vi "test1.vi"() -> ()   [LabVIEW 2020]
uses:
  <vilib>/Analysis/NI_AALBase.lvlib
  <vilib>/numeric/Random Number (Range) I64.vi
  <vilib>/DAQmx/create/channels.llb/DAQmx Create Channel (AI-Voltage-Basic).vi
  <vilib>/DAQmx/configure/timing.llb/DAQmx Timing (Implicit).vi
panel:
  in  "Terminate":bool
  in  "Choose image":bool
  out "XY Graph 3":cluster{"X":dbl[], "Y":dbl[]}[](graph)
  out "fit radius 3":dbl=0.3
  out "fit x-offset 3":dbl=0.1
  out "fit y-offset 3":dbl=0.2
  out "fit x-offset 2":dbl=0.1
  out "fit y-offset 2":dbl=0.2
  out "fit radius 2":dbl=0.3
  out "XY Graph 2":cluster{"X":dbl[], "Y":dbl[]}[](graph)
  out "Array 2":dbl[][](array[numeric])
  out "Time Stamp 2":timestamp format="%<%.6X\n%x>T"
  out "Time Stamp":timestamp format="%<%.6X\n%x>T"
  in  "x-offset":dbl=0.1
  in  "y-offset":dbl=0.2
  in  "radius":dbl=0.3
  in  "noise sigma":dbl=0.021 format="%.4f"
  out "XY Graph":cluster{"X":dbl[], "Y":dbl[]}[](graph)
  out "fit radius":dbl=0.3
  out "fit x-offset":dbl=0.1
  out "fit y-offset":dbl=0.2
  in  "loop terminate 2":bool
  out "led 2":bool
  in  "semaphore button":bool
  in  "semaphore terminate":bool
  out "led 1":bool
  out "Numeric 4":i32
  out "Cluster 3":cluster{"Numeric":dbl, "Numeric 2":dbl}
  out "Numeric 3":i32
  out "Numeric 2":i32
  out "Array":dbl[](array[numeric])
  out "Cluster 2":cluster{"Numeric 2":dbl, "Numeric 3":dbl}
  out "Cluster":cluster{"Numeric 2":dbl, "Numeric 3":dbl}
  in  "while terminate":bool
  out "cursor busy":bool
  in  "Ring":u16(ring) items=["12321"=0, "234"=1232, "343"=34343]
  out "Numeric":dbl
  in  "Cancel Button":bool
  in  "sw 3":bool
  in  "sw 2":bool
  out "Boolean 2":bool
  in  "sw":bool
  out "Boolean":bool
  out "num3":i32
  out "res":i32
  out "num2":i32
  out "num1":i32
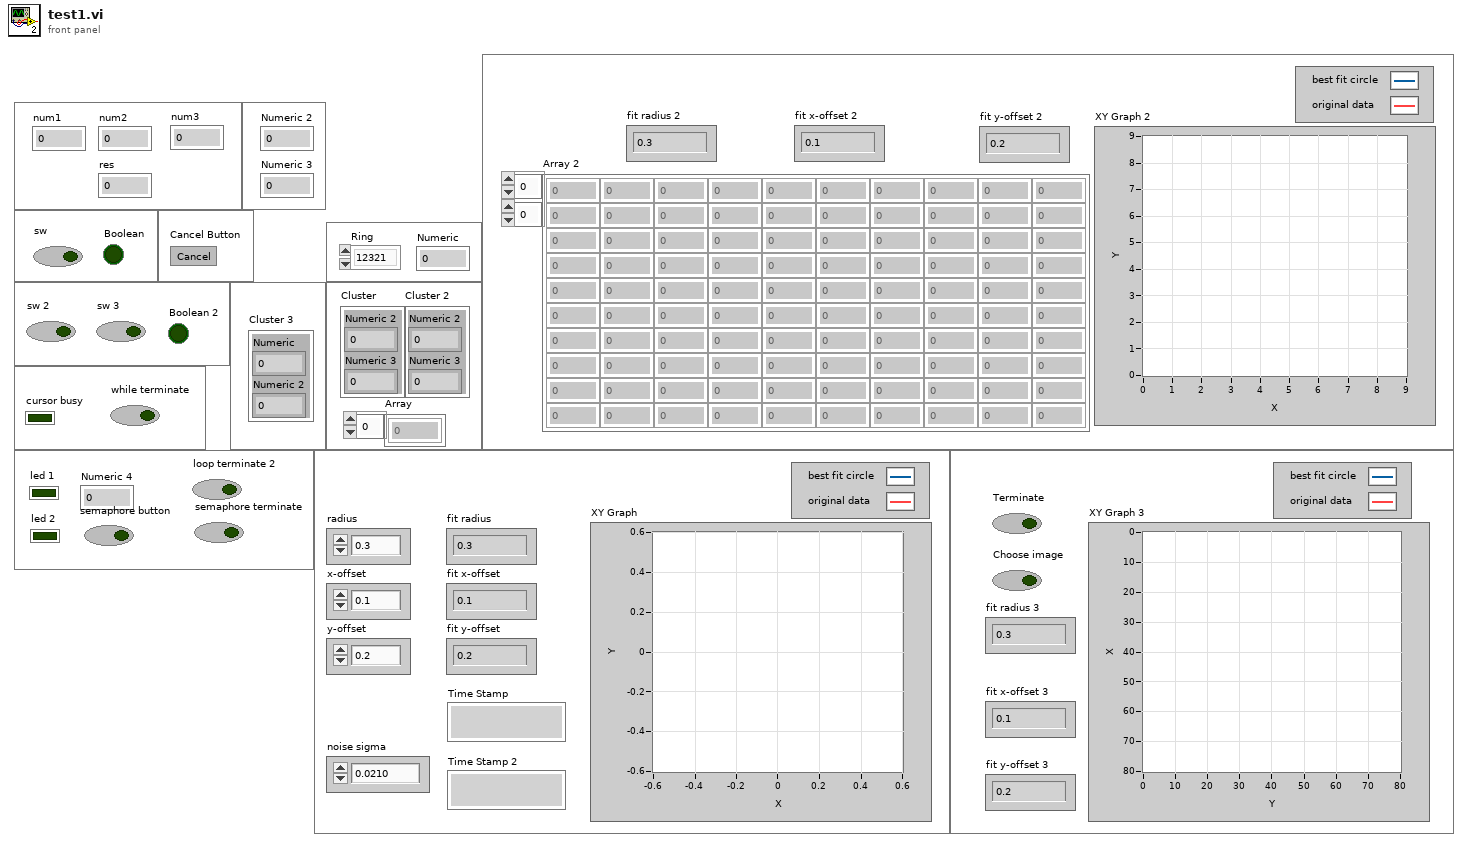
[diagram p1: front panel]
types:
  T1 = typedef "imagedata.ctl" = cluster{"image type":i32, "image depth":i32, "image":u8[], "mask":u8[], "colors":u32[], "Rectangle":cluster{"left":i16, "top":i16, "right":i16, "bottom":i16}}
  T2 = typedef "Semaphore RefNum" = refnum<k1>
  T3 = cluster{"[0]":i32, "[1]":i32, "[2]":i32, "[3]":i32, "[4]":i32, "[5]":i32, "[6]":i32, "[7]":i32, "[8]":i32}
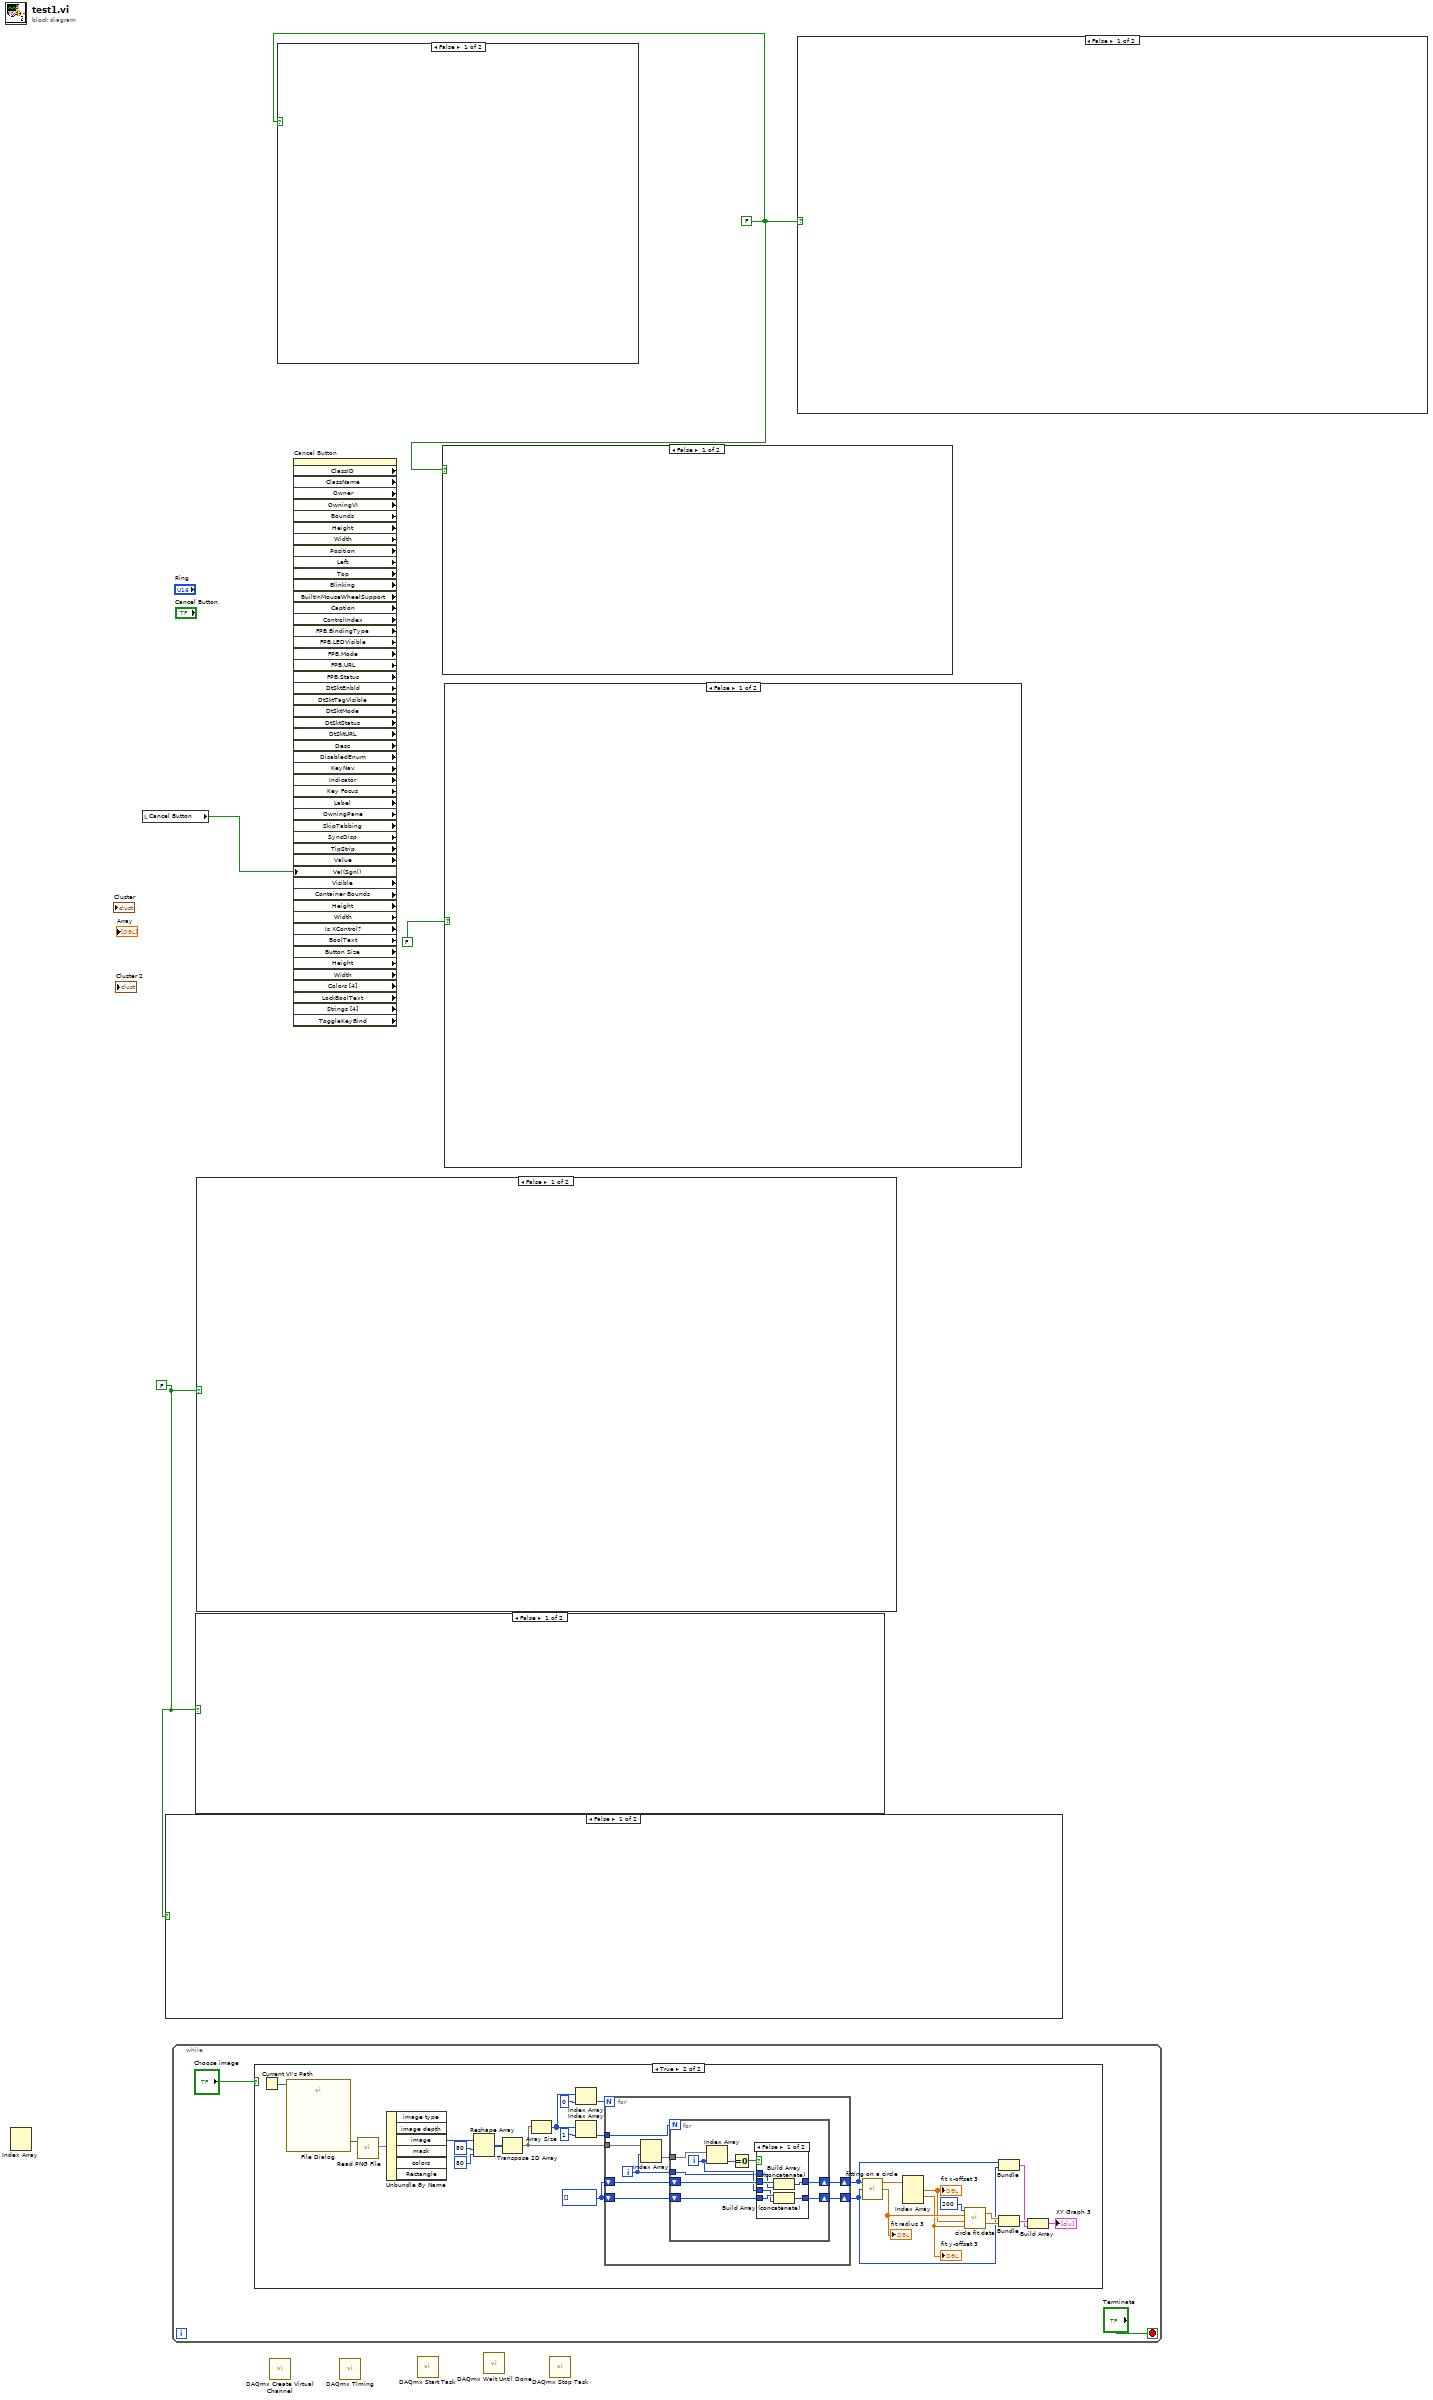
[diagram p0: block diagram]
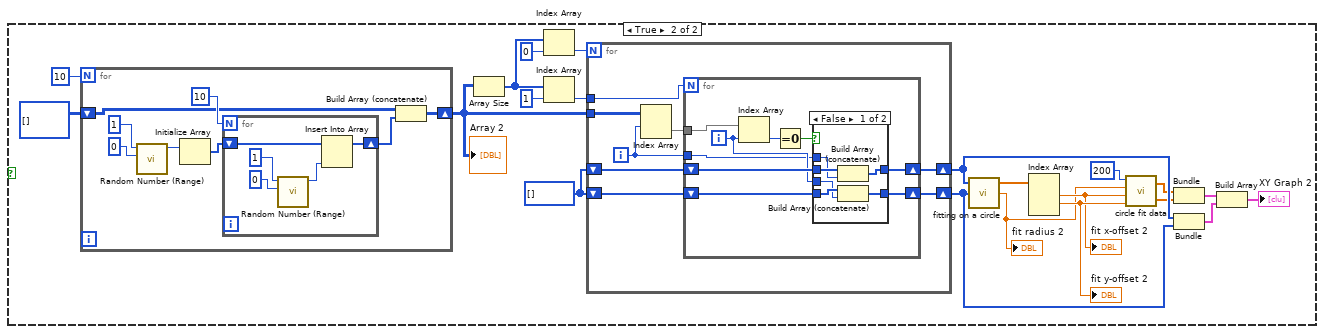
[diagram p4: hidden frame]
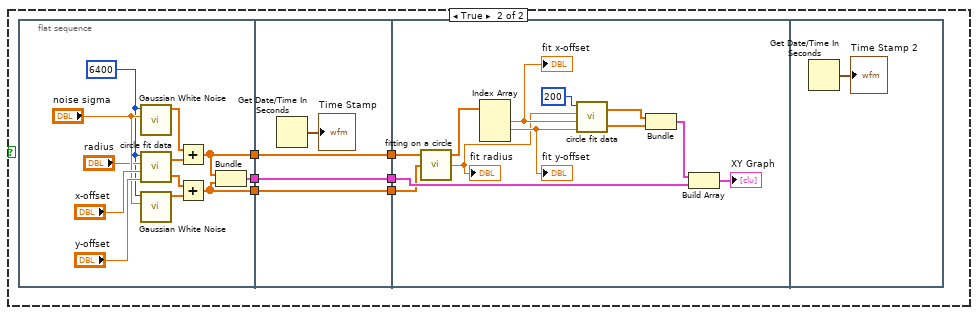
[diagram p6: hidden frame]
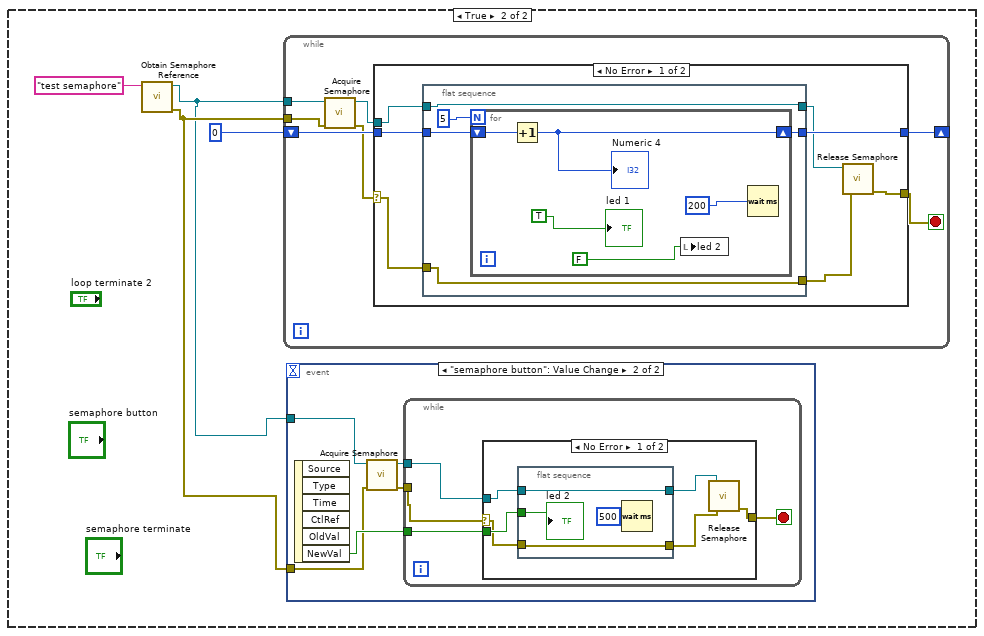
[diagram p7: hidden frame]
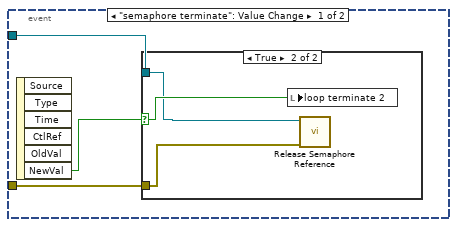
[diagram p8: hidden frame]
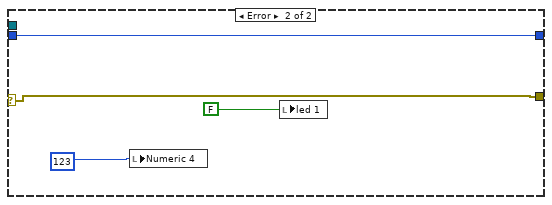
[diagram p11: hidden frame]
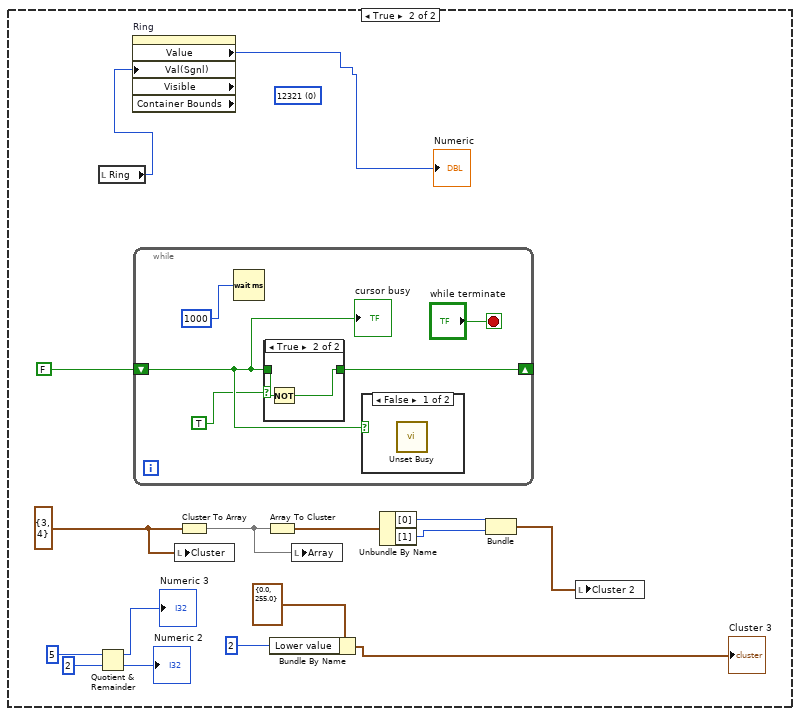
[diagram p12: hidden frame]
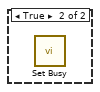
[diagram p14: hidden frame]
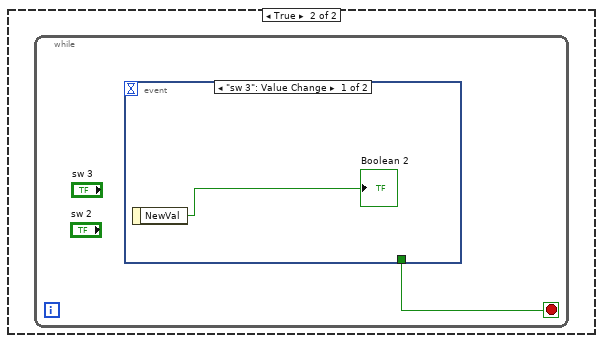
[diagram p15: hidden frame]
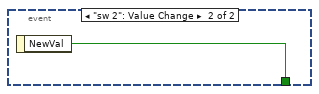
[diagram p16: hidden frame]
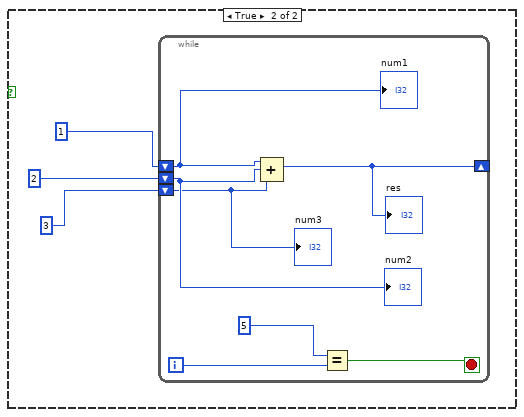
[diagram p17: hidden frame]
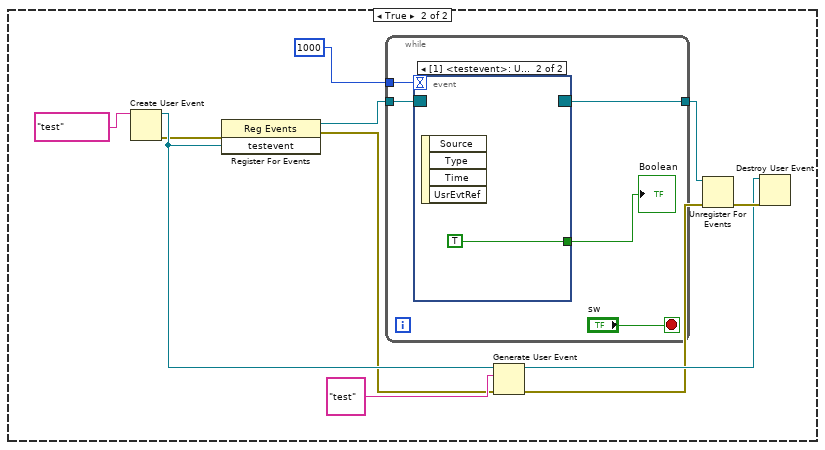
[diagram p18: hidden frame]
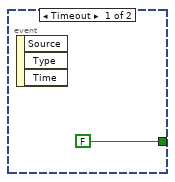
[diagram p19: hidden frame]
diagram:
  w1 = FALSE
  w4 = FALSE
  n1 = Index Array() -> ()  [unwired: 3 in, 2 out]
  n2 = local read "Cancel Button"() -> (w3:bool)
  n3 = case shown="False" w1 {
    frame False {
    }
    frame True {
      w7 = i32[] []
      n4 = for {
        N: 10 -> [_]
        shift-right: [w57] -> w21
        shift-left: i32[][] [] -> [w56]
        n5 = call-poly <vilib>:"Random Number (Range).vi"("lower bound (-100)"=0, "upper bound (100)"=1) -> ("number"=w53:i64)  [unwired: 9 in]
        n6 = Initialize Array(w53) -> (w52:i64[])  [unwired: 1 in]
        n7 = for {
          N: 10 -> [_]
          shift-right: [w59] -> w51
          shift-left: w52 -> [w60]
          n8 = call-poly <vilib>:"Random Number (Range).vi"("lower bound (-100)"=0, "upper bound (100)"=1) -> ("number"=w61:i64)  [unwired: 9 in]
          n9 = Insert Into Array(array=w60, new element=w61) -> (w59:i64[])  [unwired: 1 in]
        }
        n10 = Build Array (concatenate)(w56, w51) -> (w57:i64[][])
      }
      "Array 2" <- w21
      n11 = Array Size(array=w21) -> (size(s)=w25:i32[])
      n12 = Index Array(array=w25, index=0) -> (element=w23:i32)
      n13 = Index Array(array=w25, index=1) -> (element=w24:i32)
      n14 = for {
        N: w23 -> [_]
        tunnel: w24 -> [w33]
        shift-right: [w27] -> w15
        shift-left: w7 -> [w32]
        shift-right: [w26] -> w22
        shift-left: w7 -> [w31]
        tunnel: w21 -> [w30]
        i -> [w28]
        n15 = Index Array(array=w30, index (row)=w28) -> (element=w29:i64[])  [unwired: 1 in]
        n16 = for {
          N: w33 -> [_]
          shift-right: [w34] -> w27
          shift-left: w32 -> [w39]
          shift-right: [w38] -> w26
          shift-left: w31 -> [w37]
          tunnel: w29 -> [w42]
          tunnel: w28 -> [w35]
          i -> [w36]
          n17 = Index Array(array=w42, index=w36) -> (element=w41:i64)
          n18 = Equal To 0?(x=w41) -> (x = 0?=w40:bool)
          n19 = case shown="False" w40 {
            tunnel: w39 -> [w48 w50]
            tunnel: [w47 w49] -> w38
            tunnel: w37 -> [w46 w49]
            tunnel: w36 -> [w45 _]
            tunnel: w35 -> [w44 _]
            tunnel: [w43 w50] -> w34
            frame False {
              n20 = Build Array (concatenate)(w48, w44) -> (w43:i32[])
              n21 = Build Array (concatenate)(w46, w45) -> (w47:i32[])
            }
            frame True {
            }
          }
        }
      }
      n22 = call "fitting on a circle.vi"("Y"=w22, "X"=w15) -> ("r"=w13:dbl, "x0, y0"=w14:dbl[])  [unwired: 1 in, 1 out]
      "fit radius 2" <- w13
      n23 = Index Array(array=w14) -> (element #1=w17:dbl, element #2=w18:dbl)  [unwired: 3 in, 1 out]
      "fit x-offset 2" <- w17
      "fit y-offset 2" <- w18
      n24 = call "circle fit data.vi"("y-offset (b)"=w18, "x-offset (a)"=w17, "radius"=w13, "samples"=200) -> ("Y"=w12:dbl[], "X"=w11:dbl[])
      n25 = Bundle("X"=w11, "Y"=w12) -> (w20:cluster{"X":dbl[], "Y":dbl[]})  [unwired: 1 in]
      n26 = Bundle(w15, w22) -> (w19:cluster{i32[], i32[]})  [unwired: 1 in]
      n27 = Build Array(w20, w19) -> (→"XY Graph 2":cluster{"X":dbl[], "Y":dbl[]}[])
    }
  }
  n28 = while {
    stop <- "Terminate" stop-if-true
    n29 = case shown="True" "Choose image" {
      frame False {
      }
      frame True {
        w91 = i32[] []
        n30 = Current VI's Path() -> (path=w69:path)
        n31 = call "File Dialog"("start path"=w69) -> ("selected path"=w70:path)  [unwired: 11 in, 3 out]
        n32 = call <vilib>:"Read PNG File.vi"("path to PNG file"=w70) -> ("image data"=w74:T1)  [unwired: 8 in, 2 out]
        n33 = Unbundle By Name(w74) -> ("image"=w73:u8[])  [unwired: 5 out]
        n34 = Reshape Array(w73, 80, 80) -> (w68:u8[][])
        n35 = Transpose 2D Array(2D array=w68) -> (transposed array=w67:u8[][])
        n36 = Array Size(array=w67) -> (size(s)=w75:i32[])
        n37 = Index Array(array=w75, index=0) -> (element=w77:i32)
        n38 = Index Array(array=w75, index=1) -> (element=w76:i32)
        n39 = for {
          N: w77 -> [_]
          tunnel: w76 -> [w99]
          shift-right: [w93] -> w83
          shift-left: w91 -> [w98]
          shift-right: [w92] -> w78
          shift-left: w91 -> [w97]
          tunnel: w67 -> [w96]
          i -> [w94]
          n40 = Index Array(array=w96, index (row)=w94) -> (element=w95:u8[])  [unwired: 1 in]
          n41 = for {
            N: w99 -> [_]
            shift-right: [w100] -> w93
            shift-left: w98 -> [w105]
            shift-right: [w104] -> w92
            shift-left: w97 -> [w103]
            tunnel: w95 -> [w108]
            tunnel: w94 -> [w101]
            i -> [w102]
            n42 = Index Array(array=w108, index=w102) -> (element=w107:u8)
            n43 = Equal To 0?(x=w107) -> (x = 0?=w106:bool)
            n44 = case shown="False" w106 {
              tunnel: w105 -> [w114 w116]
              tunnel: [w113 w115] -> w104
              tunnel: w103 -> [w112 w115]
              tunnel: w102 -> [w111 _]
              tunnel: w101 -> [w110 _]
              tunnel: [w109 w116] -> w100
              frame False {
                n45 = Build Array (concatenate)(w114, w110) -> (w109:i32[])
                n46 = Build Array (concatenate)(w112, w111) -> (w113:i32[])
              }
              frame True {
              }
            }
          }
        }
        n47 = call "fitting on a circle.vi"("Y"=w78, "X"=w83) -> ("r"=w85:dbl, "x0, y0"=w84:dbl[])  [unwired: 1 in, 1 out]
        "fit radius 3" <- w85
        n48 = Index Array(array=w84) -> (element #1=w81:dbl, element #2=w80:dbl)  [unwired: 3 in, 1 out]
        "fit x-offset 3" <- w81
        "fit y-offset 3" <- w80
        n49 = call "circle fit data.vi"("y-offset (b)"=w80, "x-offset (a)"=w81, "radius"=w85, "samples"=200) -> ("Y"=w86:dbl[], "X"=w87:dbl[])
        n50 = Bundle(w83, w78) -> (w66:cluster{i32[], i32[]})  [unwired: 1 in]
        n51 = Bundle("X"=w87, "Y"=w86) -> (w79:cluster{"X":dbl[], "Y":dbl[]})  [unwired: 1 in]
        n52 = Build Array(w79, w66) -> (→"XY Graph 3":cluster{"X":dbl[], "Y":dbl[]}[])
      }
    }
  }
  n53 = case shown="False" w1 {
    frame False {
    }
    frame True {
      n54 = flat-sequence {
        tunnel: [w125] -> w122
        tunnel: [w124] -> w121
        tunnel: [w123] -> w120
        tunnel: [w137] -> w119
        tunnel: w122 -> [w137]
        tunnel: [w136] -> w118
        tunnel: w121 -> [w136]
        tunnel: [w135] -> w117
        tunnel: w120 -> [w135]
        tunnel: w119 -> [w141]
        tunnel: w118 -> [w140]
        tunnel: w117 -> [w139]
        frame #0 {
          w126 = 6400 ("samples")
          n55 = call <vilib>:"Gaussian White Noise.vi"("standard deviation"="noise sigma", "samples"=w126) -> ("Gaussian noise pattern"=w132:dbl[])  [unwired: 8 in, 1 out]
          n56 = call "circle fit data.vi"("y-offset (b)"="y-offset", "x-offset (a)"="x-offset", "radius"="radius", "samples"=w126) -> ("Y"=w128:dbl[], "X"=w127:dbl[])
          n57 = call <vilib>:"Gaussian White Noise.vi"("standard deviation"="noise sigma", "samples"=w126) -> ("Gaussian noise pattern"=w131:dbl[])  [unwired: 8 in, 1 out]
          n58 = Add(x=w132, y=w127) -> (x+y=w123:dbl[])
          n59 = Add(x=w128, y=w131) -> (x+y=w124:dbl[])
          n60 = Bundle(w123, w124) -> (w125:cluster{dbl[], dbl[]})  [unwired: 1 in]
        }
        frame #1 {
          n61 = Get Date/Time In Seconds() -> (seconds since 1Jan1904=→"Time Stamp":timestamp)
        }
        frame #2 {
          n62 = call "fitting on a circle.vi"("Y"=w140, "X"=w139) -> ("r"=w143:dbl, "x0, y0"=w142:dbl[])  [unwired: 1 in, 1 out]
          "fit radius" <- w143
          n63 = Index Array(array=w142) -> (element #1=w149:dbl, element #2=w150:dbl)  [unwired: 3 in, 1 out]
          "fit x-offset" <- w149
          "fit y-offset" <- w150
          n64 = call "circle fit data.vi"("y-offset (b)"=w150, "x-offset (a)"=w149, "radius"=w143, "samples"=200) -> ("Y"=w146:dbl[], "X"=w145:dbl[])
          n65 = Bundle("X"=w145, "Y"=w146) -> (w148:cluster{"X":dbl[], "Y":dbl[]})  [unwired: 1 in]
          n66 = Build Array(w148, w141) -> (→"XY Graph":cluster{"X":dbl[], "Y":dbl[]}[])
        }
        frame #3 {
          n67 = Get Date/Time In Seconds() -> (seconds since 1Jan1904=→"Time Stamp 2":timestamp)
        }
      }
    }
  }
  n68 = case shown="False" w1 {
    frame False {
    }
    frame True {
      n69 = call <vilib>:"Obtain Semaphore Reference.vi"("name (unnamed)"="test semaphore") -> ("error out"=w155:errorcluster, "semaphore"=w154:T2)  [unwired: 4 in, 1 out]
      n70 = while {
        shift-right: [w185] -> _
        shift-left: 0 -> [w186]
        tunnel: w154 -> [w188]
        tunnel: w155 -> [w187]
        stop <- w182 stop-if-true
        n71 = call <vilib>:"Acquire Semaphore.vi"("error in (no error)"=w187, "semaphore"=w188) -> ("error out"=w184:errorcluster, "semaphore out"=w183:T2)  [unwired: 3 in, 1 out]
        n72 = case shown="No Error" w184 {
          selector: w184 -> [w193 w206]
          tunnel: w186 -> [w195 w209]
          tunnel: [w194 w209] -> w185
          tunnel: w183 -> [w191 _]
          tunnel: [w189 w206] -> w182
          frame No Error {
            n73 = flat-sequence {
              tunnel: [w199] -> w194
              tunnel: [w197] -> w192
              tunnel: [w196] -> w190
              tunnel: w195 -> [w200]
              tunnel: w193 -> [w197]
              tunnel: w191 -> [w196]
              frame #0 {
                n74 = for {
                  N: 5 -> [_]
                  shift-right: [w203] -> w199
                  shift-left: w200 -> [w204]
                  n75 = Increment(x=w204) -> (x+1=w203:i32)
                  "Numeric 4" <- w203
                  n76 = local write "led 2"(FALSE) -> ()
                  n77 = Wait (ms)(milliseconds to wait=200) -> ()  [unwired: 1 out]
                  "led 1" <- TRUE
                }
              }
            }
            n78 = call <vilib>:"Release Semaphore.vi"("error in (no error)"=w192, "semaphore"=w190) -> ("error out"=w189:errorcluster)  [unwired: 4 in, 1 out]
          }
          frame Error {
            n79 = local write "Numeric 4"(123) -> ()
            n80 = local write "led 1"(FALSE) -> ()
          }
        }
      }
      n81 = event shown="[1] \"semaphore button\": Value Change" {
        selector: _ -> [_ _]
        dyn-events: _ -> [_ _]
        timeout: _ -> [_ _]
        tunnel: w154 -> [w157 w164]
        tunnel: w155 -> [w156 w165]
        event "semaphore terminate": Value Change {
          n82 = event-data() -> ("NewVal"=w158:bool)  [unwired: 1 in, 5 out]
          n83 = case shown="True" w158 {
            selector: w158 -> [_ w161]
            tunnel: w157 -> [_ w160]
            tunnel: w156 -> [_ w159]
            frame False {
            }
            frame True {
              n84 = local write "loop terminate 2"(w161) -> ()
              n85 = call <vilib>:"Release Semaphore Reference.vi"("error in (no error)"=w159, "semaphore"=w160) -> ()  [unwired: 8 in, 2 out]
            }
          }
        }
        event "semaphore button": Value Change {
          n86 = event-data() -> ("NewVal"=w166:bool)  [unwired: 1 in, 5 out]
          n87 = call <vilib>:"Acquire Semaphore.vi"("error in (no error)"=w165, "semaphore"=w164) -> ("error out"=w163:errorcluster, "semaphore out"=w162:T2)  [unwired: 3 in, 1 out]
          n88 = while {
            tunnel: w166 -> [w170]
            tunnel: w163 -> [w168]
            tunnel: w162 -> [w167]
            stop <- w169 stop-if-true
            n89 = case shown="No Error" w168 {
              selector: w168 -> [w173 w181]
              tunnel: w170 -> [w176 _]
              tunnel: w167 -> [w175 _]
              tunnel: [w171 w181] -> w169
              frame No Error {
                n90 = flat-sequence {
                  tunnel: [w178] -> w174
                  tunnel: [w177] -> w172
                  tunnel: w176 -> [w180]
                  tunnel: w175 -> [w178]
                  tunnel: w173 -> [w177]
                  frame #0 {
                    n91 = Wait (ms)(milliseconds to wait=500) -> ()  [unwired: 1 out]
                    "led 2" <- w180
                  }
                }
                n92 = call <vilib>:"Release Semaphore.vi"("error in (no error)"=w172, "semaphore"=w174) -> ("error out"=w171:errorcluster)  [unwired: 4 in, 1 out]
              }
              frame Error {
              }
            }
          }
        }
      }
    }
  }
  n93 = call-poly <vilib>:"DAQmx Create Virtual Channel.vi"() -> ()  [unwired: 14 in, 2 out]
  n94 = case shown="False" w4 {
    frame False {
    }
    frame True {
      n95 = while {
        shift-right: [w216] -> _
        shift-left: 1 -> [w215]
        shift-left: 2 -> [w214]
        shift-left: 3 -> [w213]
        i -> [w218]
        stop <- w217 stop-if-true
        n96 = Compound Arithmetic op=ADD(w215, w214, w213) -> (w216:i32)
        "res" <- w216
        n97 = Equal?(x=5, y=w218) -> (x = y?=w217:bool)
        "num2" <- w214
        "num1" <- w215
        "num3" <- w213
      }
    }
  }
  n98 = property on="Cancel Button" class="Bool (strict)" props=["ClassID", "ClassName", "Owner", "OwningVI", "Bounds", "Height", "Width", "Position", "Left", "Top", "Blinking", "BuiltInMouseWheelSupport", "Caption", "ControlIndex", "FPB.BindingType", "FPB.LEDVisible", "FPB.Mode", "FPB.URL", "FPB.Status", "DtSktEnbld", "DtSktTagVisible", "DtSktMode", "DtSktStatus", "DtSktURL", "Desc", "DisabledEnum", "KeyNav", "Indicator", "Key Focus", "Label", "OwningPane", "SkipTabbing", "SyncDisp", "TipStrip", "Value", "Val(Sgnl)", "Visible", "Container Bounds", "Height", "Width", "Is XControl?", "BoolText", "Button Size", "Height", "Width", "Colors [4]", "LockBoolText", "Strings [4]", "ToggleKeyBind"]("Val(Sgnl)"=w3) -> ()  [unwired: 2 in, 50 out]
  n99 = call-poly <vilib>:"DAQmx Timing.vi"() -> ()  [unwired: 14 in, 2 out]
  n100 = call <vilib>:"DAQmx Start Task.vi"() -> ()  [unwired: 14 in, 2 out]
  n101 = case shown="False" w4 {
    frame False {
    }
    frame True {
      n102 = while {
        stop <- w220 stop-if-true
        n103 = event shown="[0] \"sw 3\": Value Change" {
          selector: _ -> [_ _]
          dyn-events: _ -> [_ _]
          timeout: _ -> [_ _]
          tunnel: [_ w222] -> w220
          event "sw 3": Value Change {
            n104 = event-data() -> ("NewVal"=→"Boolean 2":bool)  [unwired: 1 in]
          }
          event "sw 2": Value Change {
            n105 = event-data() -> ("NewVal"=w222:bool)  [unwired: 1 in]
          }
        }
      }
    }
  }
  n106 = case shown="False" FALSE {
    frame False {
    }
    frame True {
      w227 = cluster{i32, i32} {3, 4}
      (unwired) u16 0 items=["12321"=0, "234"=1232, "343"=34343]
      n107 = Quotient & Remainder(x=5, y=2) -> (x-y*floor(x/y)=→"Numeric 3":i32, floor(x/y)=→"Numeric 2":i32)
      n108 = local read "Ring"() -> (w228:u16)
      n109 = property on="Ring" class="Ring (strict)" props=["Value", "Val(Sgnl)", "Visible", "Container Bounds"]("Val(Sgnl)"=w228) -> ("Value"=→"Numeric":u16)  [unwired: 2 in, 4 out]
      n110 = while {
        shift-right: [w243] -> _
        shift-left: FALSE -> [w241]
        stop <- "while terminate" stop-if-true
        n111 = Wait (ms)(milliseconds to wait=1000) -> ()  [unwired: 1 out]
        n112 = case shown="True" TRUE {
          tunnel: [w244 w246] -> w243
          tunnel: w241 -> [w244 w245]
          frame False {
          }
          frame True {
            n113 = Not(x=w245) -> (.not. x?=w246:bool)
          }
        }
        n114 = case shown="False" w241 {
          frame False {
            n115 = call <vilib>:"Unset Busy.vi"() -> ()  [unwired: 11 in, 1 out]
          }
          frame True {
            n116 = call <vilib>:"Set Busy.vi"() -> ()  [unwired: 10 in, 2 out]
          }
        }
        "cursor busy" <- w241
      }
      n117 = local write "Cluster"(w227) -> ()
      n118 = Cluster To Array(cluster=w227) -> (array=w230:i32[])
      n119 = Array To Cluster(array=w230) -> (cluster=w237:T3)
      n120 = Bundle By Name(cluster=cluster{"Lower value":sgl, "Upper value":sgl} {"Lower value"=0.0, "Upper value"=255.0} ("Threshold Limits"), "Lower value"=2) -> (→"Cluster 3":cluster{"Lower value":sgl, "Upper value":sgl})
      n121 = local write "Array"(w230) -> ()
      n122 = Unbundle By Name(w237) -> ("[0]"=w236:i32, "[1]"=w235:i32)
      n123 = Bundle("[0]"=w236, "[1]"=w235) -> (w229:cluster{"[0]":i32, "[1]":i32})  [unwired: 1 in]
      n124 = local write "Cluster 2"(w229) -> ()
    }
  }
  n125 = call <vilib>:"DAQmx Wait Until Done.vi"() -> ()  [unwired: 14 in, 2 out]
  n126 = call <vilib>:"DAQmx Stop Task.vi"() -> ()  [unwired: 14 in, 2 out]
  n127 = case shown="False" w4 {
    frame False {
    }
    frame True {
      n128 = Create User Event(user event datatype="test" ("testevent")) -> (user event=w257:refnum<user-event>, error out=w253:errorcluster)  [unwired: 1 in]
      n129 = register-events(error in=w253, w257) -> (reference out=w252:refnum<event-registration>, error out=w251:errorcluster)  [unwired: 1 in]
      n130 = while {
        tunnel: w252 -> [w262]
        tunnel: 1000 -> [w261]
        tunnel: [w259] -> w247
        stop <- "sw" stop-if-true
        n131 = event shown="[1] <testevent>: User Event" {
          selector: w262 -> [_ _]
          dyn-events: [_ _] -> w259
          timeout: w261 -> [_ _]
          tunnel: [FALSE TRUE] -> w260
          event Timeout {
            n132 = event-data() -> ()  [unwired: 1 in, 3 out]
          }
          event User Event {
            n133 = event-data() -> ()  [unwired: 1 in, 4 out]
          }
        }
        "Boolean" <- w260
      }
      n134 = Generate User Event(user event=w257, event data cluster="test", error in=w251) -> (user event out=w254:refnum<user-event>, error out=w250:errorcluster)  [unwired: 1 in]
      n135 = Unregister For Events(event registration refnum=w247, error in=w250) -> (error out=w255:errorcluster)
      n136 = Destroy User Event(user event=w254, error in=w255) -> ()  [unwired: 1 out]
    }
  }
